vi "Led_Memory_ BOUAZZOUNI.vi"() -> ()   [LabVIEW 2019]
uses:
  <vilib>/numeric/Random Number (Range) I64.vi
  <vilib>/numeric/sub_Random U32.vi
panel:
  out "Jeu":string
  out "?":string
  out "Barre de Vie":dbl(slide) scale=0.0..3.0
  out "LVL2":bool
  out "LVL5":bool
  out "LVL4":bool
  out "LVL3":bool
  out "LVL1":bool
  out "Boolean 11":bool
  out "Boolean 10":bool
  out "Boolean 9":bool
  out "Boolean 8":bool
  out "Boolean 7":bool
  out "Boolean 6":bool
  out "Boolean 5":bool
  out "Boolean 4":bool
  out "Boolean 3":bool
  in  "état de LED  11":bool
  in  "état de LED  10":bool
  in  "état de LED 9":bool
  in  "état de LED 8":bool
  in  "état de LED 7":bool
  in  "état de LED 6":bool
  in  "état de LED 5":bool
  in  "Pour BT11":bool
  in  "Pour BT9":bool
  in  "Pour BT10":bool
  in  "Pour BT8":bool
  in  "Pour BT6":bool
  in  "Pour BT7":bool
  in  "Pour BT5":bool
  in  "Pour BT3":bool
  in  "Pour BT4":bool
  out "Score":dbl
  out "Faux :(":bool
  in  "état de LED 4":bool
  in  "état de LED 3":bool
  out "Correct :)":bool
  in  "stop 2":bool
  in  "Start Button":bool
  in  "stop":bool
  # "Jeu mémoire de LED"
  # "PC"
  # "Toi"
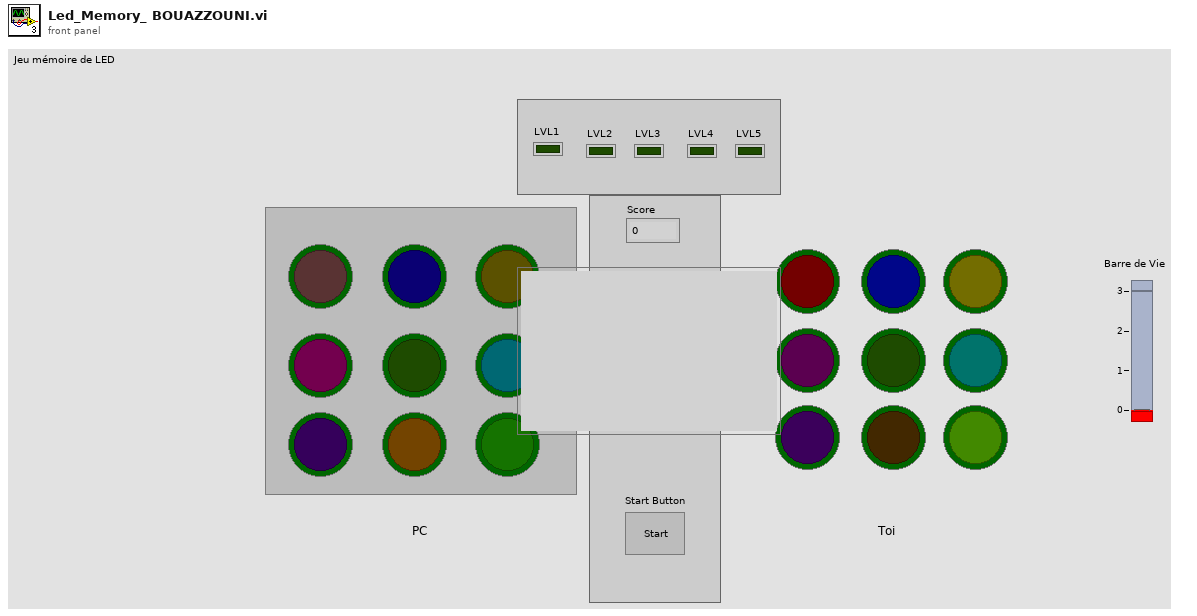
[diagram p1: front panel]
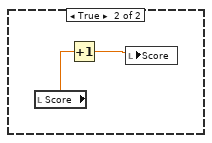
[diagram p5: hidden frame]
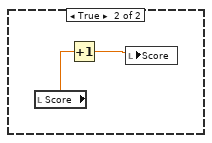
[diagram p7: hidden frame]
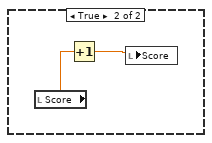
[diagram p9: hidden frame]
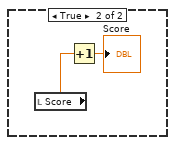
[diagram p11: hidden frame]
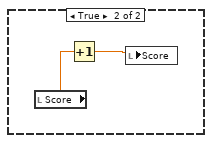
[diagram p13: hidden frame]
diagram:
  n1 = while {
    stop <- "stop" stop-if-true
    w7 = FALSE
    n2 = property on="Jeu" class="Str"("Visible"=TRUE) -> ()  [unwired: 2 in, 2 out]
    n3 = local write "Boolean 3"(w7) -> ()
    n4 = local write "Boolean 4"(w7) -> ()
    n5 = local write "Boolean 6"(w7) -> ()
    n6 = local write "Boolean 7"(w7) -> ()
    n7 = local write "Boolean 8"(w7) -> ()
    n8 = local write "Boolean 9"(w7) -> ()
    n9 = local write "Boolean 10"(w7) -> ()
    n10 = local write "Boolean 10"(w7) -> ()
    n11 = local write "état de LED 3"(w7) -> ()
    n12 = local write "état de LED 4"(w7) -> ()
    n13 = local write "état de LED 5"(w7) -> ()
    n14 = local write "état de LED 6"(w7) -> ()
    n15 = local write "état de LED 7"(w7) -> ()
    n16 = local write "état de LED 8"(w7) -> ()
    n17 = local write "état de LED 9"(w7) -> ()
    n18 = local write "état de LED  10"(w7) -> ()
    n19 = local write "état de LED  11"(w7) -> ()
    n20 = local write "LVL1"(w7) -> ()
    n21 = local write "LVL2"(w7) -> ()
    n22 = local write "LVL3"(w7) -> ()
    n23 = local write "LVL4"(w7) -> ()
    n24 = local write "LVL5"(w7) -> ()
    n25 = local write "Correct :)"(w7) -> ()
    n26 = local write "Faux :("(w7) -> ()
    n27 = local write "Score"(0) -> ()
    n28 = property on="stop" class="Bool"("Visible"=FALSE) -> ()  [unwired: 2 in, 2 out]
    n29 = property on="stop 2" class="Bool"("Visible"=FALSE) -> ()  [unwired: 2 in, 2 out]
    n30 = property class="Str"("Visible"=FALSE) -> ()  [unwired: 2 in, 2 out]
    n31 = case shown="True" "Start Button" {
      frame False {
      }
      frame True {
        n32 = while {
          stop <- "stop 2" stop-if-true
          n33 = local read "Barre de Vie"() -> (w21:dbl)
          n34 = local read "Barre de Vie"() -> (w38:dbl)
          n35 = local read "Score"() -> (w50:dbl)
          n36 = Less?(x=w50, y=2) -> (x < y?=w36:bool)
          n37 = property on="Jeu" class="Str"("Visible"=FALSE) -> ()  [unwired: 2 in, 2 out]
          n38 = Greater?(x=w21, y=0) -> (0:w35:bool)
          n39 = Less Or Equal?(x=w38, y=0) -> (x <= y?=w39:bool)
          n40 = And(x=w36, y=w35) -> (x .and. y?=w34:bool)
          n41 = case shown="True" w39 {
            frame False {
            }
            frame True {
              n42 = property class="Str"("Visible"=TRUE) -> ()  [unwired: 2 in, 2 out]
              "?" <- "\n   Game Over"
            }
          }
          n43 = case shown="True" w34 {
            frame False {
            }
            frame True {
              n44 = flat-sequence {
                frame #0 {
                  w344 = FALSE
                  n45 = call-poly <vilib>:"Random Number (Range).vi"("lower bound (-100)"=1, "upper bound (100)"=9) -> ("number"=w358:i64)  [unwired: 9 in]
                  n46 = Equal?(x=w358, y=1) -> (x = y?=w367:bool)
                  "Boolean 3" <- w367
                  n47 = local write "état de LED 3"(w367) -> ()
                  n48 = Equal?(x=w358, y=2) -> (x = y?=w366:bool)
                  "Boolean 4" <- w366
                  n49 = local write "état de LED 4"(w366) -> ()
                  n50 = Equal?(x=w358, y=3) -> (x = y?=w357:bool)
                  "Boolean 5" <- w357
                  n51 = local write "état de LED 5"(w357) -> ()
                  n52 = Equal?(x=w358, y=4) -> (x = y?=w356:bool)
                  "Boolean 6" <- w356
                  n53 = local write "état de LED 6"(w356) -> ()
                  n54 = Wait (ms)(milliseconds to wait=3000) -> ()  [unwired: 1 out]
                  n55 = Equal?(x=w358, y=5) -> (x = y?=w355:bool)
                  "Boolean 7" <- w355
                  n56 = local write "état de LED 7"(w355) -> ()
                  n57 = Equal?(x=w358, y=6) -> (x = y?=w354:bool)
                  "Boolean 8" <- w354
                  n58 = local write "état de LED 8"(w354) -> ()
                  n59 = Equal?(x=w358, y=7) -> (x = y?=w346:bool)
                  "Boolean 9" <- w346
                  n60 = local write "état de LED 9"(w346) -> ()
                  n61 = Equal?(x=w358, y=8) -> (x = y?=w353:bool)
                  "Boolean 10" <- w353
                  n62 = local write "état de LED  10"(w353) -> ()
                  n63 = Equal?(x=w358, y=9) -> (x = y?=w352:bool)
                  "Boolean 11" <- w352
                  n64 = local write "état de LED  11"(w352) -> ()
                  n65 = property on="Pour BT3" class="Bool (strict)" props=["Visible", "Container Bounds"]("Visible"=w344) -> ()  [unwired: 2 in, 3 out]
                  n66 = property on="Pour BT4" class="Bool (strict)" props=["Visible", "Container Bounds"]("Visible"=w344) -> ()  [unwired: 2 in, 3 out]
                  n67 = property on="Pour BT5" class="Bool (strict)" props=["Visible", "Container Bounds"]("Visible"=w344) -> ()  [unwired: 2 in, 3 out]
                  n68 = property on="Pour BT6" class="Bool (strict)" props=["Visible", "Container Bounds"]("Visible"=w344) -> ()  [unwired: 2 in, 3 out]
                  n69 = property on="Pour BT7" class="Bool (strict)" props=["Visible", "Container Bounds"]("Visible"=w344) -> ()  [unwired: 2 in, 3 out]
                  n70 = property on="Pour BT8" class="Bool (strict)" props=["Visible", "Container Bounds"]("Visible"=w344) -> ()  [unwired: 2 in, 3 out]
                  n71 = property on="Pour BT11" class="Bool (strict)" props=["Visible", "Container Bounds"]("Visible"=w344) -> ()  [unwired: 2 in, 3 out]
                  n72 = property on="Pour BT9" class="Bool (strict)" props=["Visible", "Container Bounds"]("Visible"=w344) -> ()  [unwired: 2 in, 3 out]
                  n73 = property on="Pour BT10" class="Bool (strict)" props=["Visible", "Container Bounds"]("Visible"=w344) -> ()  [unwired: 2 in, 3 out]
                  "LVL1" <- TRUE
                  "LVL3" <- FALSE
                  "LVL4" <- FALSE
                  "LVL5" <- FALSE
                  "LVL2" <- FALSE
                }
                frame #1 {
                  w372 = TRUE
                  w373 = FALSE
                  n74 = Wait (ms)(milliseconds to wait=3000) -> ()  [unwired: 1 out]
                  n75 = local write "Boolean 3"(w373) -> ()
                  n76 = local write "Boolean 4"(w373) -> ()
                  n77 = local write "Boolean 5"(w373) -> ()
                  n78 = local write "Boolean 6"(w373) -> ()
                  n79 = local write "Boolean 7"(w373) -> ()
                  n80 = local write "Boolean 8"(w373) -> ()
                  n81 = local write "Boolean 9"(w373) -> ()
                  n82 = local write "Boolean 10"(w373) -> ()
                  n83 = local write "Boolean 11"(w373) -> ()
                  n84 = property on="Pour BT3" class="Bool (strict)" props=["Visible", "Container Bounds"]("Visible"=w372) -> ()  [unwired: 2 in, 3 out]
                  n85 = property on="Pour BT4" class="Bool (strict)" props=["Visible", "Container Bounds"]("Visible"=w372) -> ()  [unwired: 2 in, 3 out]
                  n86 = property on="Pour BT5" class="Bool (strict)" props=["Visible", "Container Bounds"]("Visible"=w372) -> ()  [unwired: 2 in, 3 out]
                  n87 = property on="Pour BT6" class="Bool (strict)" props=["Visible", "Container Bounds"]("Visible"=w372) -> ()  [unwired: 2 in, 3 out]
                  n88 = property on="Pour BT7" class="Bool (strict)" props=["Visible", "Container Bounds"]("Visible"=w372) -> ()  [unwired: 2 in, 3 out]
                  n89 = property on="Pour BT8" class="Bool (strict)" props=["Visible", "Container Bounds"]("Visible"=w372) -> ()  [unwired: 2 in, 3 out]
                  n90 = property on="Pour BT11" class="Bool (strict)" props=["Visible", "Container Bounds"]("Visible"=w372) -> ()  [unwired: 2 in, 3 out]
                  n91 = property on="Pour BT9" class="Bool (strict)" props=["Visible", "Container Bounds"]("Visible"=w372) -> ()  [unwired: 2 in, 3 out]
                  n92 = property on="Pour BT10" class="Bool (strict)" props=["Visible", "Container Bounds"]("Visible"=w372) -> ()  [unwired: 2 in, 3 out]
                }
                frame #2 {
                  w375 = FALSE
                  n93 = Wait (ms)(milliseconds to wait=1) -> ()  [unwired: 1 out]
                  n94 = Equal?(x="état de LED  11", y="Pour BT11") -> (x = y?=w378:bool)
                  n95 = Equal?(x="état de LED 6", y="Pour BT6") -> (x = y?=w389:bool)
                  n96 = Equal?(x="état de LED  10", y="Pour BT10") -> (x = y?=w385:bool)
                  n97 = Equal?(x="état de LED 7", y="Pour BT7") -> (x = y?=w388:bool)
                  n98 = Equal?(x="état de LED 9", y="Pour BT9") -> (x = y?=w386:bool)
                  n99 = Equal?(x="état de LED 8", y="Pour BT8") -> (x = y?=w387:bool)
                  n100 = Equal?(x="état de LED 5", y="Pour BT5") -> (x = y?=w390:bool)
                  n101 = Equal?(x="état de LED 4", y="Pour BT4") -> (x = y?=w391:bool)
                  n102 = Equal?(x="état de LED 3", y="Pour BT3") -> (x = y?=w406:bool)
                  n103 = And(x=w406, y=w391) -> (x .and. y?=w384:bool)
                  n104 = And(x=w390, y=w389) -> (x .and. y?=w383:bool)
                  n105 = And(x=w388, y=w387) -> (x .and. y?=w382:bool)
                  n106 = And(x=w386, y=w385) -> (x .and. y?=w381:bool)
                  n107 = And(x=w384, y=w383) -> (x .and. y?=w380:bool)
                  n108 = And(x=w382, y=w381) -> (x .and. y?=w379:bool)
                  n109 = And(x=w380, y=w379) -> (x .and. y?=w377:bool)
                  n110 = property on="état de LED 3" class="Bool (strict)"("Visible"=w375) -> ()  [unwired: 2 in, 2 out]
                  n111 = property on="état de LED 4" class="Bool (strict)"("Visible"=w375) -> ()  [unwired: 2 in, 2 out]
                  n112 = property on="état de LED 5" class="Bool (strict)"("Visible"=w375) -> ()  [unwired: 2 in, 2 out]
                  n113 = property on="état de LED 6" class="Bool (strict)"("Visible"=w375) -> ()  [unwired: 2 in, 2 out]
                  n114 = property on="état de LED 7" class="Bool (strict)"("Visible"=w375) -> ()  [unwired: 2 in, 2 out]
                  n115 = property on="état de LED 8" class="Bool (strict)"("Visible"=w375) -> ()  [unwired: 2 in, 2 out]
                  n116 = property on="état de LED 9" class="Bool (strict)"("Visible"=w375) -> ()  [unwired: 2 in, 2 out]
                  n117 = property on="état de LED  10" class="Bool (strict)"("Visible"=w375) -> ()  [unwired: 2 in, 2 out]
                  n118 = property on="état de LED  11" class="Bool (strict)"("Visible"=w375) -> ()  [unwired: 2 in, 2 out]
                  n119 = And(x=w377, y=w378) -> (x .and. y?=w376:bool)
                  n120 = local write "Correct :)"(w376) -> ()
                }
                frame #3 {
                  w412 = FALSE
                  n121 = local read "Correct :)"() -> (w413:bool)
                  "Correct :)" <- w413
                  n122 = Wait (ms)(milliseconds to wait=1000) -> ()  [unwired: 1 out]
                  n123 = Not(x=w413) -> (.not. x?=→"Faux :(":bool)
                  n124 = case shown="False" w413 {
                    frame False {
                      n125 = local read "Barre de Vie"() -> (w417:dbl)
                      n126 = Decrement(x=w417) -> (x-1=w416:dbl)
                      n127 = local write "Barre de Vie"(w416) -> ()
                    }
                    frame True {
                      n128 = local read "Score"() -> (w418:dbl)
                      n129 = Increment(x=w418) -> (x+1=→"Score":dbl)
                    }
                  }
                  n130 = local write "Pour BT10"(w412) -> ()
                  n131 = local write "Pour BT11"(w412) -> ()
                  n132 = local write "Pour BT3"(w412) -> ()
                  n133 = local write "Pour BT4"(w412) -> ()
                  n134 = local write "Pour BT5"(w412) -> ()
                  n135 = local write "Pour BT6"(w412) -> ()
                  n136 = local write "Pour BT7"(w412) -> ()
                  n137 = local write "Pour BT8"(w412) -> ()
                  n138 = local write "Pour BT9"(w412) -> ()
                }
                frame #4 {
                  w420 = FALSE
                  n139 = local write "Correct :)"(w420) -> ()
                  n140 = local write "Faux :("(w420) -> ()
                  n141 = Wait (ms)(milliseconds to wait=1) -> ()  [unwired: 1 out]
                }
              }
            }
          }
          n142 = Wait (ms)(milliseconds to wait=1) -> ()  [unwired: 1 out]
          n143 = local read "Barre de Vie"() -> (w19:dbl)
          n144 = local read "Score"() -> (w46:dbl)
          n145 = Greater?(x=w19, y=0) -> (0:w33:bool)
          n146 = Equal?(x=w46, y=2) -> (x = y?=w32:bool)
          n147 = And(x=w32, y=w33) -> ()  [unwired: 1 out]
          n148 = case shown="True" w32 {
            frame False {
            }
            frame True {
              (unwired) FALSE
              n149 = flat-sequence {
                frame #0 {
                  w470 = FALSE
                  n150 = call-poly <vilib>:"Random Number (Range).vi"("lower bound (-100)"=1, "upper bound (100)"=9) -> ("number"=w430:i64)  [unwired: 9 in]
                  n151 = Equal?(x=w430, y=1) -> (x = y?=w457:bool)
                  n152 = call-poly <vilib>:"Random Number (Range).vi"("lower bound (-100)"=10, "upper bound (100)"=18) -> ("number"=w424:i64)  [unwired: 9 in]
                  n153 = Equal?(x=10, y=w424) -> (x = y?=w455:bool)
                  n154 = Exclusive Or(1:w455, 2:w457) -> (0:w456:bool)
                  n155 = Wait (ms)(milliseconds to wait=3000) -> ()  [unwired: 1 out]
                  n156 = local write "Boolean 3"(w456) -> ()
                  n157 = local write "état de LED 3"(w456) -> ()
                  n158 = Equal?(x=w430, y=2) -> (x = y?=w459:bool)
                  n159 = Equal?(x=w424, y=11) -> (x = y?=w458:bool)
                  n160 = Exclusive Or(1:w458, 2:w459) -> (0:w460:bool)
                  n161 = local write "état de LED 4"(w460) -> ()
                  n162 = local write "Boolean 4"(w460) -> ()
                  n163 = Equal?(x=w430, y=3) -> (x = y?=w452:bool)
                  n164 = Equal?(x=w424, y=12) -> (x = y?=w451:bool)
                  n165 = Exclusive Or(1:w451, 2:w452) -> (0:w450:bool)
                  n166 = local write "état de LED 5"(w450) -> ()
                  n167 = local write "Boolean 5"(w450) -> ()
                  n168 = Equal?(x=w430, y=4) -> (x = y?=w448:bool)
                  n169 = Equal?(x=w424, y=13) -> (x = y?=w447:bool)
                  n170 = Exclusive Or(1:w447, 2:w448) -> (0:w446:bool)
                  n171 = local write "état de LED 6"(w446) -> ()
                  n172 = local write "Boolean 6"(w446) -> ()
                  n173 = local write "LVL1"(FALSE) -> ()
                  n174 = Equal?(x=w430, y=5) -> (x = y?=w444:bool)
                  n175 = Equal?(x=14, y=w424) -> (x = y?=w443:bool)
                  n176 = Exclusive Or(1:w443, 2:w444) -> (0:w442:bool)
                  n177 = local write "LVL2"(TRUE) -> ()
                  n178 = local write "Boolean 7"(w442) -> ()
                  n179 = local write "état de LED 7"(w442) -> ()
                  n180 = Equal?(x=w430, y=6) -> (x = y?=w439:bool)
                  n181 = Equal?(x=15, y=w424) -> (x = y?=w441:bool)
                  n182 = local write "LVL3"(FALSE) -> ()
                  n183 = Exclusive Or(1:w441, 2:w439) -> (0:w438:bool)
                  n184 = local write "état de LED 8"(w438) -> ()
                  n185 = local write "Boolean 8"(w438) -> ()
                  n186 = local write "LVL4"(FALSE) -> ()
                  n187 = Equal?(x=w430, y=7) -> (x = y?=w435:bool)
                  n188 = Equal?(x=16, y=w424) -> (x = y?=w437:bool)
                  n189 = Exclusive Or(1:w437, 2:w435) -> (0:w434:bool)
                  n190 = local write "LVL5"(FALSE) -> ()
                  n191 = local write "Boolean 9"(w434) -> ()
                  n192 = local write "état de LED 9"(w434) -> ()
                  n193 = Equal?(x=17, y=w424) -> (x = y?=w433:bool)
                  n194 = Equal?(x=w430, y=8) -> (x = y?=w429:bool)
                  n195 = Exclusive Or(1:w433, 2:w429) -> (0:w431:bool)
                  n196 = local write "Boolean 10"(w431) -> ()
                  n197 = local write "état de LED  10"(w431) -> ()
                  n198 = Equal?(x=w430, y=9) -> (x = y?=w426:bool)
                  n199 = Equal?(x=18, y=w424) -> (x = y?=w428:bool)
                  n200 = Exclusive Or(1:w428, 2:w426) -> (0:w425:bool)
                  n201 = local write "état de LED  11"(w425) -> ()
                  n202 = local write "Boolean 11"(w425) -> ()
                  n203 = property on="Pour BT3" class="Bool (strict)" props=["Visible", "Container Bounds"]("Visible"=w470) -> ()  [unwired: 2 in, 3 out]
                  n204 = property on="Pour BT4" class="Bool (strict)" props=["Visible", "Container Bounds"]("Visible"=w470) -> ()  [unwired: 2 in, 3 out]
                  n205 = property on="Pour BT5" class="Bool (strict)" props=["Visible", "Container Bounds"]("Visible"=w470) -> ()  [unwired: 2 in, 3 out]
                  n206 = property on="Pour BT6" class="Bool (strict)" props=["Visible", "Container Bounds"]("Visible"=w470) -> ()  [unwired: 2 in, 3 out]
                  n207 = property on="Pour BT7" class="Bool (strict)" props=["Visible", "Container Bounds"]("Visible"=w470) -> ()  [unwired: 2 in, 3 out]
                  n208 = property on="Pour BT8" class="Bool (strict)" props=["Visible", "Container Bounds"]("Visible"=w470) -> ()  [unwired: 2 in, 3 out]
                  n209 = property on="Pour BT11" class="Bool (strict)" props=["Visible", "Container Bounds"]("Visible"=w470) -> ()  [unwired: 2 in, 3 out]
                  n210 = property on="Pour BT9" class="Bool (strict)" props=["Visible", "Container Bounds"]("Visible"=w470) -> ()  [unwired: 2 in, 3 out]
                  n211 = property on="Pour BT10" class="Bool (strict)" props=["Visible", "Container Bounds"]("Visible"=w470) -> ()  [unwired: 2 in, 3 out]
                }
                frame #1 {
                  w482 = TRUE
                  w483 = FALSE
                  n212 = Wait (ms)(milliseconds to wait=3000) -> ()  [unwired: 1 out]
                  n213 = local write "Boolean 3"(w483) -> ()
                  n214 = local write "Boolean 4"(w483) -> ()
                  n215 = local write "Boolean 5"(w483) -> ()
                  n216 = local write "Boolean 6"(w483) -> ()
                  n217 = local write "Boolean 7"(w483) -> ()
                  n218 = local write "Boolean 8"(w483) -> ()
                  n219 = local write "Boolean 9"(w483) -> ()
                  n220 = local write "Boolean 10"(w483) -> ()
                  n221 = local write "Boolean 11"(w483) -> ()
                  n222 = property on="Pour BT3" class="Bool (strict)" props=["Visible", "Container Bounds"]("Visible"=w482) -> ()  [unwired: 2 in, 3 out]
                  n223 = property on="Pour BT4" class="Bool (strict)" props=["Visible", "Container Bounds"]("Visible"=w482) -> ()  [unwired: 2 in, 3 out]
                  n224 = property on="Pour BT5" class="Bool (strict)" props=["Visible", "Container Bounds"]("Visible"=w482) -> ()  [unwired: 2 in, 3 out]
                  n225 = property on="Pour BT6" class="Bool (strict)" props=["Visible", "Container Bounds"]("Visible"=w482) -> ()  [unwired: 2 in, 3 out]
                  n226 = property on="Pour BT7" class="Bool (strict)" props=["Visible", "Container Bounds"]("Visible"=w482) -> ()  [unwired: 2 in, 3 out]
                  n227 = property on="Pour BT8" class="Bool (strict)" props=["Visible", "Container Bounds"]("Visible"=w482) -> ()  [unwired: 2 in, 3 out]
                  n228 = property on="Pour BT11" class="Bool (strict)" props=["Visible", "Container Bounds"]("Visible"=w482) -> ()  [unwired: 2 in, 3 out]
                  n229 = property on="Pour BT9" class="Bool (strict)" props=["Visible", "Container Bounds"]("Visible"=w482) -> ()  [unwired: 2 in, 3 out]
                  n230 = property on="Pour BT10" class="Bool (strict)" props=["Visible", "Container Bounds"]("Visible"=w482) -> ()  [unwired: 2 in, 3 out]
                }
                frame #2 {
                  n231 = local read "état de LED  10"() -> (w488:bool)
                  n232 = local read "état de LED 8"() -> (w492:bool)
                  n233 = local read "état de LED 9"() -> (w490:bool)
                  n234 = local read "Pour BT8"() -> (w491:bool)
                  n235 = local read "Pour BT9"() -> (w489:bool)
                  n236 = local read "Pour BT10"() -> (w487:bool)
                  n237 = local read "état de LED 6"() -> (w496:bool)
                  n238 = local read "Pour BT11"() -> (w485:bool)
                  n239 = local read "Pour BT6"() -> (w495:bool)
                  n240 = local read "état de LED  11"() -> (w486:bool)
                  n241 = local read "état de LED 7"() -> (w494:bool)
                  n242 = local read "état de LED 5"() -> (w498:bool)
                  n243 = local read "Pour BT7"() -> (w493:bool)
                  n244 = local read "Pour BT4"() -> (w499:bool)
                  n245 = local read "Pour BT5"() -> (w497:bool)
                  n246 = local read "état de LED 4"() -> (w500:bool)
                  n247 = local read "Pour BT3"() -> (w501:bool)
                  n248 = local read "état de LED 3"() -> (w502:bool)
                  n249 = Wait (ms)(milliseconds to wait=1) -> ()  [unwired: 1 out]
                  n250 = Equal?(x=w486, y=w485) -> (x = y?=w505:bool)
                  n251 = Equal?(x=w496, y=w495) -> (x = y?=w516:bool)
                  n252 = Equal?(x=w488, y=w487) -> (x = y?=w512:bool)
                  n253 = Equal?(x=w494, y=w493) -> (x = y?=w515:bool)
                  n254 = Equal?(x=w490, y=w489) -> (x = y?=w513:bool)
                  n255 = Equal?(x=w492, y=w491) -> (x = y?=w514:bool)
                  n256 = Equal?(x=w498, y=w497) -> (x = y?=w517:bool)
                  n257 = Equal?(x=w500, y=w499) -> (x = y?=w518:bool)
                  n258 = Equal?(x=w502, y=w501) -> (x = y?=w519:bool)
                  n259 = And(x=w519, y=w518) -> (x .and. y?=w511:bool)
                  n260 = And(x=w517, y=w516) -> (x .and. y?=w510:bool)
                  n261 = And(x=w515, y=w514) -> (x .and. y?=w509:bool)
                  n262 = And(x=w513, y=w512) -> (x .and. y?=w508:bool)
                  n263 = And(x=w511, y=w510) -> (x .and. y?=w507:bool)
                  n264 = And(x=w509, y=w508) -> (x .and. y?=w506:bool)
                  n265 = And(x=w507, y=w506) -> (x .and. y?=w504:bool)
                  n266 = And(x=w504, y=w505) -> (x .and. y?=w503:bool)
                  n267 = local write "Correct :)"(w503) -> ()
                }
                frame #3 {
                  w523 = FALSE
                  n268 = local read "Correct :)"() -> (w521:bool)
                  n269 = Wait (ms)(milliseconds to wait=1000) -> ()  [unwired: 1 out]
                  n270 = Not(x=w521) -> (.not. x?=w522:bool)
                  n271 = local write "Correct :)"(w521) -> ()
                  n272 = local write "Faux :("(w522) -> ()
                  n273 = case shown="False" w521 {
                    frame False {
                      n274 = local read "Barre de Vie"() -> (w525:dbl)
                      n275 = Decrement(x=w525) -> (x-1=w526:dbl)
                      n276 = local write "Barre de Vie"(w526) -> ()
                    }
                    frame True {
                      n277 = local read "Score"() -> (w528:dbl)
                      n278 = Increment(x=w528) -> (x+1=w527:dbl)
                      n279 = local write "Score"(w527) -> ()
                    }
                  }
                  n280 = local write "Pour BT10"(w523) -> ()
                  n281 = local write "Pour BT11"(w523) -> ()
                  n282 = local write "Pour BT3"(w523) -> ()
                  n283 = local write "Pour BT4"(w523) -> ()
                  n284 = local write "Pour BT5"(w523) -> ()
                  n285 = local write "Pour BT6"(w523) -> ()
                  n286 = local write "Pour BT7"(w523) -> ()
                  n287 = local write "Pour BT8"(w523) -> ()
                  n288 = local write "Pour BT9"(w523) -> ()
                }
                frame #4 {
                  w529 = FALSE
                  n289 = local write "Correct :)"(w529) -> ()
                  n290 = local write "Faux :("(w529) -> ()
                  n291 = Wait (ms)(milliseconds to wait=1) -> ()  [unwired: 1 out]
                }
              }
              n292 = local write "LVL2"(TRUE) -> ()
              n293 = Wait (ms)(milliseconds to wait=5000) -> ()  [unwired: 1 out]
            }
          }
          n294 = local read "Barre de Vie"() -> (w17:dbl)
          n295 = local read "Score"() -> (w44:dbl)
          n296 = Greater?(x=w17, y=0) -> (0:w31:bool)
          n297 = Equal?(x=w44, y=3) -> (x = y?=w30:bool)
          n298 = And(x=w30, y=w31) -> (x .and. y?=w29:bool)
          n299 = case shown="True" w29 {
            frame False {
            }
            frame True {
              n300 = flat-sequence {
                frame #0 {
                  w276 = FALSE
                  n301 = call-poly <vilib>:"Random Number (Range).vi"("lower bound (-100)"=1, "upper bound (100)"=9) -> ("number"=w212:i64)  [unwired: 9 in]
                  n302 = call-poly <vilib>:"Random Number (Range).vi"("lower bound (-100)"=1, "upper bound (100)"=9) -> ("number"=w213:i64)  [unwired: 9 in]
                  n303 = Equal?(x=1, y=w213) -> (x = y?=w275:bool)
                  n304 = Wait (ms)(milliseconds to wait=3000) -> ()  [unwired: 1 out]
                  n305 = call-poly <vilib>:"Random Number (Range).vi"("lower bound (-100)"=1, "upper bound (100)"=9) -> ("number"=w283:i64)  [unwired: 9 in]
                  n306 = Equal?(x=w283, y=1) -> (x = y?=w273:bool)
                  n307 = Exclusive Or(1:w275, 2:w273) -> (0:w271:bool)
                  n308 = Equal?(x=1, y=w212) -> (x = y?=w270:bool)
                  n309 = Exclusive Or(1:w270, 2:w271) -> (0:w269:bool)
                  n310 = local write "Boolean 3"(w269) -> ()
                  n311 = local write "état de LED 3"(w269) -> ()
                  n312 = Equal?(x=2, y=w213) -> (x = y?=w268:bool)
                  n313 = Equal?(x=w283, y=2) -> (x = y?=w263:bool)
                  n314 = Exclusive Or(1:w268, 2:w263) -> (0:w265:bool)
                  n315 = Equal?(x=2, y=w212) -> (x = y?=w264:bool)
                  n316 = Exclusive Or(1:w264, 2:w265) -> (0:w262:bool)
                  n317 = local write "Boolean 4"(w262) -> ()
                  n318 = local write "état de LED 4"(w262) -> ()
                  n319 = Equal?(x=3, y=w213) -> (x = y?=w261:bool)
                  n320 = Equal?(x=w283, y=3) -> (x = y?=w256:bool)
                  n321 = Exclusive Or(1:w261, 2:w256) -> (0:w258:bool)
                  n322 = Equal?(x=3, y=w212) -> (x = y?=w257:bool)
                  n323 = Exclusive Or(1:w257, 2:w258) -> (0:w255:bool)
                  n324 = local write "état de LED 5"(w255) -> ()
                  n325 = local write "Boolean 5"(w255) -> ()
                  n326 = Equal?(x=w283, y=4) -> (x = y?=w250:bool)
                  n327 = Equal?(x=4, y=w213) -> (x = y?=w254:bool)
                  n328 = Exclusive Or(1:w254, 2:w250) -> (0:w249:bool)
                  n329 = local write "Boolean 6"(w249) -> ()
                  n330 = local write "état de LED 6"(w249) -> ()
                  n331 = Equal?(x=4, y=w212) -> (x = y?=w251:bool)
                  n332 = Exclusive Or(1:w251, 2:w249) -> ()  [unwired: 1 out]
                  n333 = Equal?(x=w283, y=5) -> (x = y?=w243:bool)
                  n334 = local write "LVL1"(FALSE) -> ()
                  n335 = Equal?(x=5, y=w213) -> (x = y?=w248:bool)
                  n336 = Exclusive Or(1:w248, 2:w243) -> (0:w245:bool)
                  n337 = Equal?(x=5, y=w212) -> (x = y?=w244:bool)
                  n338 = local write "LVL2"(FALSE) -> ()
                  n339 = Exclusive Or(1:w244, 2:w245) -> (0:w242:bool)
                  n340 = local write "Boolean 7"(w242) -> ()
                  n341 = local write "état de LED 7"(w242) -> ()
                  n342 = Equal?(x=w283, y=6) -> (x = y?=w236:bool)
                  n343 = Equal?(x=6, y=w213) -> (x = y?=w241:bool)
                  n344 = local write "LVL3"(TRUE) -> ()
                  n345 = Exclusive Or(1:w241, 2:w236) -> (0:w238:bool)
                  n346 = Equal?(x=6, y=w212) -> (x = y?=w237:bool)
                  n347 = Exclusive Or(1:w237, 2:w238) -> (0:w235:bool)
                  n348 = local write "Boolean 8"(w235) -> ()
                  n349 = local write "état de LED 8"(w235) -> ()
                  n350 = local write "LVL4"(FALSE) -> ()
                  n351 = Equal?(x=w283, y=7) -> (x = y?=w229:bool)
                  n352 = Equal?(x=7, y=w213) -> (x = y?=w234:bool)
                  n353 = Exclusive Or(1:w234, 2:w229) -> (0:w231:bool)
                  n354 = local write "LVL5"(FALSE) -> ()
                  n355 = Equal?(x=7, y=w212) -> (x = y?=w230:bool)
                  n356 = Exclusive Or(1:w230, 2:w231) -> (0:w228:bool)
                  n357 = local write "Boolean 9"(w228) -> ()
                  n358 = local write "état de LED 9"(w228) -> ()
                  n359 = Equal?(x=w283, y=8) -> (x = y?=w222:bool)
                  n360 = Equal?(x=8, y=w213) -> (x = y?=w227:bool)
                  n361 = Exclusive Or(1:w227, 2:w222) -> (0:w224:bool)
                  n362 = Equal?(x=8, y=w212) -> (x = y?=w223:bool)
                  n363 = Exclusive Or(1:w223, 2:w224) -> (0:w221:bool)
                  n364 = local write "Boolean 10"(w221) -> ()
                  n365 = local write "état de LED  10"(w221) -> ()
                  n366 = Equal?(x=w283, y=9) -> (x = y?=w215:bool)
                  n367 = Equal?(x=9, y=w213) -> (x = y?=w220:bool)
                  n368 = Exclusive Or(1:w220, 2:w215) -> (0:w217:bool)
                  n369 = Equal?(x=9, y=w212) -> (x = y?=w216:bool)
                  n370 = Exclusive Or(1:w216, 2:w217) -> (0:w214:bool)
                  n371 = local write "état de LED  11"(w214) -> ()
                  n372 = local write "Boolean 11"(w214) -> ()
                  n373 = property on="Pour BT3" class="Bool (strict)" props=["Visible", "Container Bounds"]("Visible"=w276) -> ()  [unwired: 2 in, 3 out]
                  n374 = property on="Pour BT4" class="Bool (strict)" props=["Visible", "Container Bounds"]("Visible"=w276) -> ()  [unwired: 2 in, 3 out]
                  n375 = property on="Pour BT5" class="Bool (strict)" props=["Visible", "Container Bounds"]("Visible"=w276) -> ()  [unwired: 2 in, 3 out]
                  n376 = property on="Pour BT6" class="Bool (strict)" props=["Visible", "Container Bounds"]("Visible"=w276) -> ()  [unwired: 2 in, 3 out]
                  n377 = property on="Pour BT7" class="Bool (strict)" props=["Visible", "Container Bounds"]("Visible"=w276) -> ()  [unwired: 2 in, 3 out]
                  n378 = property on="Pour BT8" class="Bool (strict)" props=["Visible", "Container Bounds"]("Visible"=w276) -> ()  [unwired: 2 in, 3 out]
                  n379 = property on="Pour BT11" class="Bool (strict)" props=["Visible", "Container Bounds"]("Visible"=w276) -> ()  [unwired: 2 in, 3 out]
                  n380 = property on="Pour BT9" class="Bool (strict)" props=["Visible", "Container Bounds"]("Visible"=w276) -> ()  [unwired: 2 in, 3 out]
                  n381 = property on="Pour BT10" class="Bool (strict)" props=["Visible", "Container Bounds"]("Visible"=w276) -> ()  [unwired: 2 in, 3 out]
                }
                frame #1 {
                  w295 = TRUE
                  w296 = FALSE
                  n382 = Wait (ms)(milliseconds to wait=3000) -> ()  [unwired: 1 out]
                  n383 = local write "Boolean 3"(w296) -> ()
                  n384 = local write "Boolean 4"(w296) -> ()
                  n385 = local write "Boolean 5"(w296) -> ()
                  n386 = local write "Boolean 6"(w296) -> ()
                  n387 = local write "Boolean 7"(w296) -> ()
                  n388 = local write "Boolean 8"(w296) -> ()
                  n389 = local write "Boolean 9"(w296) -> ()
                  n390 = local write "Boolean 10"(w296) -> ()
                  n391 = local write "Boolean 11"(w296) -> ()
                  n392 = property on="Pour BT3" class="Bool (strict)" props=["Visible", "Container Bounds"]("Visible"=w295) -> ()  [unwired: 2 in, 3 out]
                  n393 = property on="Pour BT4" class="Bool (strict)" props=["Visible", "Container Bounds"]("Visible"=w295) -> ()  [unwired: 2 in, 3 out]
                  n394 = property on="Pour BT5" class="Bool (strict)" props=["Visible", "Container Bounds"]("Visible"=w295) -> ()  [unwired: 2 in, 3 out]
                  n395 = property on="Pour BT6" class="Bool (strict)" props=["Visible", "Container Bounds"]("Visible"=w295) -> ()  [unwired: 2 in, 3 out]
                  n396 = property on="Pour BT7" class="Bool (strict)" props=["Visible", "Container Bounds"]("Visible"=w295) -> ()  [unwired: 2 in, 3 out]
                  n397 = property on="Pour BT8" class="Bool (strict)" props=["Visible", "Container Bounds"]("Visible"=w295) -> ()  [unwired: 2 in, 3 out]
                  n398 = property on="Pour BT11" class="Bool (strict)" props=["Visible", "Container Bounds"]("Visible"=w295) -> ()  [unwired: 2 in, 3 out]
                  n399 = property on="Pour BT9" class="Bool (strict)" props=["Visible", "Container Bounds"]("Visible"=w295) -> ()  [unwired: 2 in, 3 out]
                  n400 = property on="Pour BT10" class="Bool (strict)" props=["Visible", "Container Bounds"]("Visible"=w295) -> ()  [unwired: 2 in, 3 out]
                }
                frame #2 {
                  n401 = local read "état de LED  10"() -> (w301:bool)
                  n402 = local read "état de LED 8"() -> (w305:bool)
                  n403 = local read "état de LED 9"() -> (w303:bool)
                  n404 = local read "Pour BT8"() -> (w304:bool)
                  n405 = local read "Pour BT9"() -> (w302:bool)
                  n406 = local read "Pour BT10"() -> (w300:bool)
                  n407 = local read "état de LED 6"() -> (w309:bool)
                  n408 = local read "Pour BT11"() -> (w298:bool)
                  n409 = local read "Pour BT6"() -> (w308:bool)
                  n410 = local read "état de LED  11"() -> (w299:bool)
                  n411 = local read "état de LED 7"() -> (w307:bool)
                  n412 = local read "état de LED 5"() -> (w311:bool)
                  n413 = local read "Pour BT7"() -> (w306:bool)
                  n414 = local read "Pour BT4"() -> (w312:bool)
                  n415 = local read "Pour BT5"() -> (w310:bool)
                  n416 = local read "état de LED 4"() -> (w313:bool)
                  n417 = local read "Pour BT3"() -> (w314:bool)
                  n418 = local read "état de LED 3"() -> (w315:bool)
                  n419 = Wait (ms)(milliseconds to wait=1) -> ()  [unwired: 1 out]
                  n420 = Equal?(x=w299, y=w298) -> (x = y?=w318:bool)
                  n421 = Equal?(x=w309, y=w308) -> (x = y?=w329:bool)
                  n422 = Equal?(x=w301, y=w300) -> (x = y?=w325:bool)
                  n423 = Equal?(x=w307, y=w306) -> (x = y?=w328:bool)
                  n424 = Equal?(x=w303, y=w302) -> (x = y?=w326:bool)
                  n425 = Equal?(x=w305, y=w304) -> (x = y?=w327:bool)
                  n426 = Equal?(x=w311, y=w310) -> (x = y?=w330:bool)
                  n427 = Equal?(x=w313, y=w312) -> (x = y?=w331:bool)
                  n428 = Equal?(x=w315, y=w314) -> (x = y?=w332:bool)
                  n429 = And(x=w332, y=w331) -> (x .and. y?=w324:bool)
                  n430 = And(x=w330, y=w329) -> (x .and. y?=w323:bool)
                  n431 = And(x=w328, y=w327) -> (x .and. y?=w322:bool)
                  n432 = And(x=w326, y=w325) -> (x .and. y?=w321:bool)
                  n433 = And(x=w324, y=w323) -> (x .and. y?=w320:bool)
                  n434 = And(x=w322, y=w321) -> (x .and. y?=w319:bool)
                  n435 = And(x=w320, y=w319) -> (x .and. y?=w317:bool)
                  n436 = And(x=w317, y=w318) -> (x .and. y?=w316:bool)
                  n437 = local write "Correct :)"(w316) -> ()
                }
                frame #3 {
                  w336 = FALSE
                  n438 = local read "Correct :)"() -> (w334:bool)
                  n439 = Wait (ms)(milliseconds to wait=1000) -> ()  [unwired: 1 out]
                  n440 = Not(x=w334) -> (.not. x?=w335:bool)
                  n441 = local write "Correct :)"(w334) -> ()
                  n442 = local write "Faux :("(w335) -> ()
                  n443 = case shown="False" w334 {
                    frame False {
                      n444 = local read "Barre de Vie"() -> (w338:dbl)
                      n445 = Decrement(x=w338) -> (x-1=w339:dbl)
                      n446 = local write "Barre de Vie"(w339) -> ()
                    }
                    frame True {
                      n447 = local read "Score"() -> (w341:dbl)
                      n448 = Increment(x=w341) -> (x+1=w340:dbl)
                      n449 = local write "Score"(w340) -> ()
                    }
                  }
                  n450 = local write "Pour BT10"(w336) -> ()
                  n451 = local write "Pour BT11"(w336) -> ()
                  n452 = local write "Pour BT3"(w336) -> ()
                  n453 = local write "Pour BT4"(w336) -> ()
                  n454 = local write "Pour BT5"(w336) -> ()
                  n455 = local write "Pour BT6"(w336) -> ()
                  n456 = local write "Pour BT7"(w336) -> ()
                  n457 = local write "Pour BT8"(w336) -> ()
                  n458 = local write "Pour BT9"(w336) -> ()
                }
                frame #4 {
                  w342 = FALSE
                  n459 = local write "Correct :)"(w342) -> ()
                  n460 = local write "Faux :("(w342) -> ()
                  n461 = Wait (ms)(milliseconds to wait=1) -> ()  [unwired: 1 out]
                }
              }
            }
          }
          n462 = local read "Barre de Vie"() -> (w15:dbl)
          n463 = local read "Score"() -> (w41:dbl)
          n464 = Greater?(x=w15, y=0) -> (0:w28:bool)
          n465 = Equal?(x=w41, y=4) -> (x = y?=w27:bool)
          n466 = And(x=w27, y=w28) -> (x .and. y?=w26:bool)
          n467 = case shown="True" w26 {
            frame False {
            }
            frame True {
              n468 = flat-sequence {
                frame #0 {
                  w131 = FALSE
                  n469 = call-poly <vilib>:"Random Number (Range).vi"("lower bound (-100)"=1, "upper bound (100)"=3) -> ("number"=w147:i64)  [unwired: 9 in]
                  n470 = Equal?(x=w147, y=1) -> (x = y?=w140:bool)
                  n471 = local write "Boolean 3"(w140) -> ()
                  n472 = local write "état de LED 3"(w140) -> ()
                  n473 = Equal?(x=w147, y=1) -> (x = y?=w139:bool)
                  n474 = local write "Boolean 4"(w139) -> ()
                  n475 = local write "état de LED 4"(w139) -> ()
                  n476 = Equal?(x=w147, y=1) -> (x = y?=w138:bool)
                  n477 = local write "Boolean 5"(w138) -> ()
                  n478 = local write "état de LED 5"(w138) -> ()
                  n479 = Equal?(x=w147, y=1) -> (x = y?=w137:bool)
                  n480 = local write "état de LED 6"(w137) -> ()
                  n481 = local write "Boolean 6"(w137) -> ()
                  n482 = Wait (ms)(milliseconds to wait=3000) -> ()  [unwired: 1 out]
                  n483 = Equal?(x=w147, y=2) -> (x = y?=w136:bool)
                  n484 = local write "LVL1"(FALSE) -> ()
                  n485 = local write "Boolean 7"(w136) -> ()
                  n486 = local write "LVL2"(FALSE) -> ()
                  n487 = local write "état de LED 7"(w136) -> ()
                  n488 = Equal?(x=w147, y=2) -> (x = y?=w135:bool)
                  n489 = local write "LVL3"(FALSE) -> ()
                  n490 = local write "Boolean 8"(w135) -> ()
                  n491 = local write "état de LED 8"(w135) -> ()
                  n492 = local write "LVL4"(TRUE) -> ()
                  n493 = Equal?(x=w147, y=2) -> (x = y?=w134:bool)
                  n494 = local write "LVL5"(FALSE) -> ()
                  n495 = local write "Boolean 9"(w134) -> ()
                  n496 = local write "état de LED 9"(w134) -> ()
                  n497 = Equal?(x=w147, y=2) -> (x = y?=w132:bool)
                  n498 = local write "Boolean 10"(w132) -> ()
                  n499 = local write "état de LED  10"(w132) -> ()
                  n500 = Equal?(x=w147, y=1) -> (x = y?=w133:bool)
                  n501 = local write "état de LED  11"(w133) -> ()
                  n502 = local write "Boolean 11"(w133) -> ()
                  n503 = property on="Pour BT3" class="Bool (strict)" props=["Visible", "Container Bounds"]("Visible"=w131) -> ()  [unwired: 2 in, 3 out]
                  n504 = property on="Pour BT4" class="Bool (strict)" props=["Visible", "Container Bounds"]("Visible"=w131) -> ()  [unwired: 2 in, 3 out]
                  n505 = property on="Pour BT5" class="Bool (strict)" props=["Visible", "Container Bounds"]("Visible"=w131) -> ()  [unwired: 2 in, 3 out]
                  n506 = property on="Pour BT6" class="Bool (strict)" props=["Visible", "Container Bounds"]("Visible"=w131) -> ()  [unwired: 2 in, 3 out]
                  n507 = property on="Pour BT7" class="Bool (strict)" props=["Visible", "Container Bounds"]("Visible"=w131) -> ()  [unwired: 2 in, 3 out]
                  n508 = property on="Pour BT8" class="Bool (strict)" props=["Visible", "Container Bounds"]("Visible"=w131) -> ()  [unwired: 2 in, 3 out]
                  n509 = property on="Pour BT11" class="Bool (strict)" props=["Visible", "Container Bounds"]("Visible"=w131) -> ()  [unwired: 2 in, 3 out]
                  n510 = property on="Pour BT9" class="Bool (strict)" props=["Visible", "Container Bounds"]("Visible"=w131) -> ()  [unwired: 2 in, 3 out]
                  n511 = property on="Pour BT10" class="Bool (strict)" props=["Visible", "Container Bounds"]("Visible"=w131) -> ()  [unwired: 2 in, 3 out]
                }
                frame #1 {
                  w159 = TRUE
                  w160 = FALSE
                  n512 = Wait (ms)(milliseconds to wait=3000) -> ()  [unwired: 1 out]
                  n513 = local write "Boolean 3"(w160) -> ()
                  n514 = local write "Boolean 4"(w160) -> ()
                  n515 = local write "Boolean 5"(w160) -> ()
                  n516 = local write "Boolean 6"(w160) -> ()
                  n517 = local write "Boolean 7"(w160) -> ()
                  n518 = local write "Boolean 8"(w160) -> ()
                  n519 = local write "Boolean 9"(w160) -> ()
                  n520 = local write "Boolean 10"(w160) -> ()
                  n521 = local write "Boolean 11"(w160) -> ()
                  n522 = property on="Pour BT3" class="Bool (strict)" props=["Visible", "Container Bounds"]("Visible"=w159) -> ()  [unwired: 2 in, 3 out]
                  n523 = property on="Pour BT4" class="Bool (strict)" props=["Visible", "Container Bounds"]("Visible"=w159) -> ()  [unwired: 2 in, 3 out]
                  n524 = property on="Pour BT5" class="Bool (strict)" props=["Visible", "Container Bounds"]("Visible"=w159) -> ()  [unwired: 2 in, 3 out]
                  n525 = property on="Pour BT6" class="Bool (strict)" props=["Visible", "Container Bounds"]("Visible"=w159) -> ()  [unwired: 2 in, 3 out]
                  n526 = property on="Pour BT7" class="Bool (strict)" props=["Visible", "Container Bounds"]("Visible"=w159) -> ()  [unwired: 2 in, 3 out]
                  n527 = property on="Pour BT8" class="Bool (strict)" props=["Visible", "Container Bounds"]("Visible"=w159) -> ()  [unwired: 2 in, 3 out]
                  n528 = property on="Pour BT11" class="Bool (strict)" props=["Visible", "Container Bounds"]("Visible"=w159) -> ()  [unwired: 2 in, 3 out]
                  n529 = property on="Pour BT9" class="Bool (strict)" props=["Visible", "Container Bounds"]("Visible"=w159) -> ()  [unwired: 2 in, 3 out]
                  n530 = property on="Pour BT10" class="Bool (strict)" props=["Visible", "Container Bounds"]("Visible"=w159) -> ()  [unwired: 2 in, 3 out]
                }
                frame #2 {
                  n531 = local read "état de LED  10"() -> (w165:bool)
                  n532 = local read "état de LED 8"() -> (w169:bool)
                  n533 = local read "état de LED 9"() -> (w167:bool)
                  n534 = local read "Pour BT8"() -> (w168:bool)
                  n535 = local read "Pour BT9"() -> (w166:bool)
                  n536 = local read "Pour BT10"() -> (w164:bool)
                  n537 = local read "état de LED 6"() -> (w173:bool)
                  n538 = local read "Pour BT11"() -> (w162:bool)
                  n539 = local read "Pour BT6"() -> (w172:bool)
                  n540 = local read "état de LED  11"() -> (w163:bool)
                  n541 = local read "état de LED 7"() -> (w171:bool)
                  n542 = local read "état de LED 5"() -> (w175:bool)
                  n543 = local read "Pour BT7"() -> (w170:bool)
                  n544 = local read "Pour BT4"() -> (w176:bool)
                  n545 = local read "Pour BT5"() -> (w174:bool)
                  n546 = local read "état de LED 4"() -> (w177:bool)
                  n547 = local read "Pour BT3"() -> (w178:bool)
                  n548 = local read "état de LED 3"() -> (w179:bool)
                  n549 = Wait (ms)(milliseconds to wait=1) -> ()  [unwired: 1 out]
                  n550 = Equal?(x=w163, y=w162) -> (x = y?=w182:bool)
                  n551 = Equal?(x=w173, y=w172) -> (x = y?=w193:bool)
                  n552 = Equal?(x=w165, y=w164) -> (x = y?=w189:bool)
                  n553 = Equal?(x=w171, y=w170) -> (x = y?=w192:bool)
                  n554 = Equal?(x=w167, y=w166) -> (x = y?=w190:bool)
                  n555 = Equal?(x=w169, y=w168) -> (x = y?=w191:bool)
                  n556 = Equal?(x=w175, y=w174) -> (x = y?=w194:bool)
                  n557 = Equal?(x=w177, y=w176) -> (x = y?=w195:bool)
                  n558 = Equal?(x=w179, y=w178) -> (x = y?=w196:bool)
                  n559 = And(x=w196, y=w195) -> (x .and. y?=w188:bool)
                  n560 = And(x=w194, y=w193) -> (x .and. y?=w187:bool)
                  n561 = And(x=w192, y=w191) -> (x .and. y?=w186:bool)
                  n562 = And(x=w190, y=w189) -> (x .and. y?=w185:bool)
                  n563 = And(x=w188, y=w187) -> (x .and. y?=w184:bool)
                  n564 = And(x=w186, y=w185) -> (x .and. y?=w183:bool)
                  n565 = And(x=w184, y=w183) -> (x .and. y?=w181:bool)
                  n566 = And(x=w181, y=w182) -> (x .and. y?=w180:bool)
                  n567 = local write "Correct :)"(w180) -> ()
                }
                frame #3 {
                  w200 = FALSE
                  n568 = local read "Correct :)"() -> (w198:bool)
                  n569 = Wait (ms)(milliseconds to wait=1000) -> ()  [unwired: 1 out]
                  n570 = Not(x=w198) -> (.not. x?=w199:bool)
                  n571 = local write "Correct :)"(w198) -> ()
                  n572 = local write "Faux :("(w199) -> ()
                  n573 = case shown="False" w198 {
                    frame False {
                      n574 = local read "Barre de Vie"() -> (w203:dbl)
                      n575 = Decrement(x=w203) -> (x-1=w202:dbl)
                      n576 = local write "Barre de Vie"(w202) -> ()
                    }
                    frame True {
                      n577 = local read "Score"() -> (w205:dbl)
                      n578 = Increment(x=w205) -> (x+1=w204:dbl)
                      n579 = local write "Score"(w204) -> ()
                    }
                  }
                  n580 = local write "Pour BT10"(w200) -> ()
                  n581 = local write "Pour BT11"(w200) -> ()
                  n582 = local write "Pour BT3"(w200) -> ()
                  n583 = local write "Pour BT4"(w200) -> ()
                  n584 = local write "Pour BT5"(w200) -> ()
                  n585 = local write "Pour BT6"(w200) -> ()
                  n586 = local write "Pour BT7"(w200) -> ()
                  n587 = local write "Pour BT8"(w200) -> ()
                  n588 = local write "Pour BT9"(w200) -> ()
                }
                frame #4 {
                  w206 = FALSE
                  n589 = local write "Correct :)"(w206) -> ()
                  n590 = local write "Faux :("(w206) -> ()
                  n591 = Wait (ms)(milliseconds to wait=1) -> ()  [unwired: 1 out]
                }
              }
            }
          }
          n592 = local read "Barre de Vie"() -> (w13:dbl)
          n593 = local read "Score"() -> (w42:dbl)
          n594 = Greater?(x=w13, y=0) -> (0:w25:bool)
          n595 = Greater Or Equal?(x=w42, y=5) -> (x >= y?=w24:bool)
          n596 = And(x=w24, y=w25) -> (x .and. y?=w23:bool)
          n597 = case shown="True" w23 {
            frame False {
            }
            frame True {
              n598 = flat-sequence {
                frame #0 {
                  w54 = FALSE
                  n599 = call-poly <vilib>:"Random Number (Range).vi"("lower bound (-100)"=1, "upper bound (100)"=2) -> ("number"=w70:i64)  [unwired: 9 in]
                  n600 = Equal?(x=w70, y=1) -> (x = y?=w63:bool)
                  n601 = local write "Boolean 3"(w63) -> ()
                  n602 = local write "état de LED 3"(w63) -> ()
                  n603 = Equal?(x=w70, y=1) -> (x = y?=w62:bool)
                  n604 = local write "Boolean 4"(w62) -> ()
                  n605 = local write "état de LED 4"(w62) -> ()
                  n606 = Equal?(x=w70, y=1) -> (x = y?=w61:bool)
                  n607 = local write "Boolean 5"(w61) -> ()
                  n608 = local write "état de LED 5"(w61) -> ()
                  n609 = Equal?(x=w70, y=1) -> (x = y?=w60:bool)
                  n610 = local write "état de LED 6"(w60) -> ()
                  n611 = local write "Boolean 6"(w60) -> ()
                  n612 = Wait (ms)(milliseconds to wait=3000) -> ()  [unwired: 1 out]
                  n613 = Equal?(x=w70, y=1) -> (x = y?=w59:bool)
                  n614 = local write "LVL1"(FALSE) -> ()
                  n615 = local write "Boolean 7"(w59) -> ()
                  n616 = local write "LVL2"(FALSE) -> ()
                  n617 = local write "état de LED 7"(w59) -> ()
                  n618 = Equal?(x=w70, y=2) -> (x = y?=w58:bool)
                  n619 = local write "LVL3"(FALSE) -> ()
                  n620 = local write "Boolean 8"(w58) -> ()
                  n621 = local write "état de LED 8"(w58) -> ()
                  n622 = local write "LVL4"(FALSE) -> ()
                  n623 = Equal?(x=w70, y=2) -> (x = y?=w57:bool)
                  n624 = local write "LVL5"(TRUE) -> ()
                  n625 = local write "Boolean 9"(w57) -> ()
                  n626 = local write "état de LED 9"(w57) -> ()
                  n627 = Equal?(x=w70, y=2) -> (x = y?=w55:bool)
                  n628 = local write "Boolean 10"(w55) -> ()
                  n629 = local write "état de LED  10"(w55) -> ()
                  n630 = Equal?(x=w70, y=2) -> (x = y?=w56:bool)
                  n631 = local write "état de LED  11"(w56) -> ()
                  n632 = local write "Boolean 11"(w56) -> ()
                  n633 = property on="Pour BT3" class="Bool (strict)" props=["Visible", "Container Bounds"]("Visible"=w54) -> ()  [unwired: 2 in, 3 out]
                  n634 = property on="Pour BT4" class="Bool (strict)" props=["Visible", "Container Bounds"]("Visible"=w54) -> ()  [unwired: 2 in, 3 out]
                  n635 = property on="Pour BT5" class="Bool (strict)" props=["Visible", "Container Bounds"]("Visible"=w54) -> ()  [unwired: 2 in, 3 out]
                  n636 = property on="Pour BT6" class="Bool (strict)" props=["Visible", "Container Bounds"]("Visible"=w54) -> ()  [unwired: 2 in, 3 out]
                  n637 = property on="Pour BT7" class="Bool (strict)" props=["Visible", "Container Bounds"]("Visible"=w54) -> ()  [unwired: 2 in, 3 out]
                  n638 = property on="Pour BT8" class="Bool (strict)" props=["Visible", "Container Bounds"]("Visible"=w54) -> ()  [unwired: 2 in, 3 out]
                  n639 = property on="Pour BT11" class="Bool (strict)" props=["Visible", "Container Bounds"]("Visible"=w54) -> ()  [unwired: 2 in, 3 out]
                  n640 = property on="Pour BT9" class="Bool (strict)" props=["Visible", "Container Bounds"]("Visible"=w54) -> ()  [unwired: 2 in, 3 out]
                  n641 = property on="Pour BT10" class="Bool (strict)" props=["Visible", "Container Bounds"]("Visible"=w54) -> ()  [unwired: 2 in, 3 out]
                }
                frame #1 {
                  w82 = TRUE
                  w83 = FALSE
                  n642 = Wait (ms)(milliseconds to wait=3000) -> ()  [unwired: 1 out]
                  n643 = local write "Boolean 3"(w83) -> ()
                  n644 = local write "Boolean 4"(w83) -> ()
                  n645 = local write "Boolean 5"(w83) -> ()
                  n646 = local write "Boolean 6"(w83) -> ()
                  n647 = local write "Boolean 7"(w83) -> ()
                  n648 = local write "Boolean 8"(w83) -> ()
                  n649 = local write "Boolean 9"(w83) -> ()
                  n650 = local write "Boolean 10"(w83) -> ()
                  n651 = local write "Boolean 11"(w83) -> ()
                  n652 = property on="Pour BT3" class="Bool (strict)" props=["Visible", "Container Bounds"]("Visible"=w82) -> ()  [unwired: 2 in, 3 out]
                  n653 = property on="Pour BT4" class="Bool (strict)" props=["Visible", "Container Bounds"]("Visible"=w82) -> ()  [unwired: 2 in, 3 out]
                  n654 = property on="Pour BT5" class="Bool (strict)" props=["Visible", "Container Bounds"]("Visible"=w82) -> ()  [unwired: 2 in, 3 out]
                  n655 = property on="Pour BT6" class="Bool (strict)" props=["Visible", "Container Bounds"]("Visible"=w82) -> ()  [unwired: 2 in, 3 out]
                  n656 = property on="Pour BT7" class="Bool (strict)" props=["Visible", "Container Bounds"]("Visible"=w82) -> ()  [unwired: 2 in, 3 out]
                  n657 = property on="Pour BT8" class="Bool (strict)" props=["Visible", "Container Bounds"]("Visible"=w82) -> ()  [unwired: 2 in, 3 out]
                  n658 = property on="Pour BT11" class="Bool (strict)" props=["Visible", "Container Bounds"]("Visible"=w82) -> ()  [unwired: 2 in, 3 out]
                  n659 = property on="Pour BT9" class="Bool (strict)" props=["Visible", "Container Bounds"]("Visible"=w82) -> ()  [unwired: 2 in, 3 out]
                  n660 = property on="Pour BT10" class="Bool (strict)" props=["Visible", "Container Bounds"]("Visible"=w82) -> ()  [unwired: 2 in, 3 out]
                }
                frame #2 {
                  n661 = local read "état de LED  10"() -> (w88:bool)
                  n662 = local read "état de LED 8"() -> (w92:bool)
                  n663 = local read "état de LED 9"() -> (w90:bool)
                  n664 = local read "Pour BT8"() -> (w91:bool)
                  n665 = local read "Pour BT9"() -> (w89:bool)
                  n666 = local read "Pour BT10"() -> (w87:bool)
                  n667 = local read "état de LED 6"() -> (w96:bool)
                  n668 = local read "Pour BT11"() -> (w85:bool)
                  n669 = local read "Pour BT6"() -> (w95:bool)
                  n670 = local read "état de LED  11"() -> (w86:bool)
                  n671 = local read "état de LED 7"() -> (w94:bool)
                  n672 = local read "état de LED 5"() -> (w98:bool)
                  n673 = local read "Pour BT7"() -> (w93:bool)
                  n674 = local read "Pour BT4"() -> (w99:bool)
                  n675 = local read "Pour BT5"() -> (w97:bool)
                  n676 = local read "état de LED 4"() -> (w100:bool)
                  n677 = local read "Pour BT3"() -> (w101:bool)
                  n678 = local read "état de LED 3"() -> (w102:bool)
                  n679 = Wait (ms)(milliseconds to wait=1) -> ()  [unwired: 1 out]
                  n680 = Equal?(x=w86, y=w85) -> (x = y?=w105:bool)
                  n681 = Equal?(x=w96, y=w95) -> (x = y?=w116:bool)
                  n682 = Equal?(x=w88, y=w87) -> (x = y?=w112:bool)
                  n683 = Equal?(x=w94, y=w93) -> (x = y?=w115:bool)
                  n684 = Equal?(x=w90, y=w89) -> (x = y?=w113:bool)
                  n685 = Equal?(x=w92, y=w91) -> (x = y?=w114:bool)
                  n686 = Equal?(x=w98, y=w97) -> (x = y?=w117:bool)
                  n687 = Equal?(x=w100, y=w99) -> (x = y?=w118:bool)
                  n688 = Equal?(x=w102, y=w101) -> (x = y?=w119:bool)
                  n689 = And(x=w119, y=w118) -> (x .and. y?=w111:bool)
                  n690 = And(x=w117, y=w116) -> (x .and. y?=w110:bool)
                  n691 = And(x=w115, y=w114) -> (x .and. y?=w109:bool)
                  n692 = And(x=w113, y=w112) -> (x .and. y?=w108:bool)
                  n693 = And(x=w111, y=w110) -> (x .and. y?=w107:bool)
                  n694 = And(x=w109, y=w108) -> (x .and. y?=w106:bool)
                  n695 = And(x=w107, y=w106) -> (x .and. y?=w104:bool)
                  n696 = And(x=w104, y=w105) -> (x .and. y?=w103:bool)
                  n697 = local write "Correct :)"(w103) -> ()
                }
                frame #3 {
                  w123 = FALSE
                  n698 = local read "Correct :)"() -> (w121:bool)
                  n699 = Wait (ms)(milliseconds to wait=1000) -> ()  [unwired: 1 out]
                  n700 = Not(x=w121) -> (.not. x?=w122:bool)
                  n701 = local write "Correct :)"(w121) -> ()
                  n702 = local write "Faux :("(w122) -> ()
                  n703 = case shown="False" w121 {
                    frame False {
                      n704 = local read "Barre de Vie"() -> (w126:dbl)
                      n705 = Decrement(x=w126) -> (x-1=w125:dbl)
                      n706 = local write "Barre de Vie"(w125) -> ()
                    }
                    frame True {
                      n707 = local read "Score"() -> (w128:dbl)
                      n708 = Increment(x=w128) -> (x+1=w127:dbl)
                      n709 = local write "Score"(w127) -> ()
                    }
                  }
                  n710 = local write "Pour BT10"(w123) -> ()
                  n711 = local write "Pour BT11"(w123) -> ()
                  n712 = local write "Pour BT3"(w123) -> ()
                  n713 = local write "Pour BT4"(w123) -> ()
                  n714 = local write "Pour BT5"(w123) -> ()
                  n715 = local write "Pour BT6"(w123) -> ()
                  n716 = local write "Pour BT7"(w123) -> ()
                  n717 = local write "Pour BT8"(w123) -> ()
                  n718 = local write "Pour BT9"(w123) -> ()
                }
                frame #4 {
                  w129 = FALSE
                  n719 = local write "Correct :)"(w129) -> ()
                  n720 = local write "Faux :("(w129) -> ()
                  n721 = Wait (ms)(milliseconds to wait=1) -> ()  [unwired: 1 out]
                }
              }
            }
          }
        }
      }
    }
    n722 = Wait (ms)(milliseconds to wait=1) -> ()  [unwired: 1 out]
    "Barre de Vie" <- 3
    "Jeu" <- "Ce jeu est un jeu de mémoire.\nAppuyer sur start pour commencer.\nLe principe du jeu est simple, des led en couleurs s'allument et tu dois les mémoriser et reproduire la même configuration des leds de ton côté !\nIl y a une barre de vie de 3 niveaux, lorsque la barre arrive à 0 le jeu s'arrête.\nLe jeu est constitué de 5 niveaux.\nPour passer d’un niveau à un autre, il faut gagner en score.\n\n                                  Bon jeu !"
  }
